vi "Get WiFi Info.vi"(8 "Error In":errorcluster, 11 "LINX Resource":T2={"IO"=enum."Remote", "Interface"=enum."Serial", "LINX Device Config"={"Interface"=enum."Serial", "COM Port"="COM13", "TCP Configuration"={"IP Address"="", "Port"=0}, "Device Family"=1, "Device ID"=1, "Device Name"="myRIO-1900", "TCP Ref"=refnum, "Channels"={"DI"=[0, 1, 2, 3, 4, 5, 6, 7, 8, 9, 10, 11, 12, 13, 14, 15, 16, 17, 18, 19, 20, 21, 22, 23, 24, 25, 26, 27, 28, 29, 30, 31, 32, 33, 34, 35, 36, 37, 38, 39, 40, 41, 42, 43, 44, 45, 46], "DO"=[0, 1, 2, 3, 4, 5, 6, 7, 8, 9, 10, 11, 12, 13, 14, 15, 16, 17, 18, 19, 20, 21, 22, 23, 24, 25, 26, 27, 28, 29, 30, 31, 32, 33, 34, 35, 36, 37, 38, 39, 40, 41, 42, 43, 44, 45, 46], "AI"=[0, 1, 2, 3, 4, 5, 6, 7, 8, 9, 10, 11], "AO"=[], "PWM"=[3, 5, 6, 9, 10], "QE"=[], "UART"=[0, 1], "I2C 2"=[0], "SPI"=[0], "CAN"=[], "Servo"=[], "AI Ref (V)"=0.0, "AI Resolution (Bits)"=0, "AO Ref (V)"=0.0, "AO Resolution (Bits)"=0}}}) -> (0 "Error Out":errorcluster, 1 "TCP Config":T1, 2 "WiFi Info":T7={"SSID"="", "IP Address"="", "Port"=0, "WIFI Security Type"=enum."WPA2 Password", "Password"=""}, 3 "LINX Resource Out":T2={"IO"=enum."Remote", "Interface"=enum."Serial", "LINX Device Config"={"Interface"=enum."Serial", "COM Port"="COM13", "TCP Configuration"={"IP Address"="", "Port"=0}, "Device Family"=1, "Device ID"=1, "Device Name"="myRIO-1900", "TCP Ref"=refnum, "Channels"={"DI"=[0, 1, 2, 3, 4, 5, 6, 7, 8, 9, 10, 11, 12, 13, 14, 15, 16, 17, 18, 19, 20, 21, 22, 23, 24, 25, 26, 27, 28, 29, 30, 31, 32, 33, 34, 35, 36, 37, 38, 39, 40, 41, 42, 43, 44, 45, 46], "DO"=[0, 1, 2, 3, 4, 5, 6, 7, 8, 9, 10, 11, 12, 13, 14, 15, 16, 17, 18, 19, 20, 21, 22, 23, 24, 25, 26, 27, 28, 29, 30, 31, 32, 33, 34, 35, 36, 37, 38, 39, 40, 41, 42, 43, 44, 45, 46], "AI"=[0, 1, 2, 3, 4, 5, 6, 7, 8, 9, 10, 11], "AO"=[], "PWM"=[3, 5, 6, 9, 10], "QE"=[], "UART"=[0, 1], "I2C 2"=[0], "SPI"=[0], "CAN"=[], "Servo"=[], "AI Ref (V)"=0.0, "AI Resolution (Bits)"=0, "AO Ref (V)"=0.0, "AO Resolution (Bits)"=0}}})   [LabVIEW 2019, in "LINXx.lvlib"]
doc: "Lists the WiFi settings currently saved on the device."
uses:
  LINXx.lvlib
  <vilib>/MakerHub/LINX/Private/Device/Type Defs/Wifi Config.ctl
  <vilib>/MakerHub/LINX/Private/Type Defs/WIFI Security Type.ctl
  <vilib>/MakerHub/LINX/Private/Type Defs/LINX Ref.ctl
  <vilib>/MakerHub/LINX/Private/Type Defs/Platform.ctl
  <vilib>/MakerHub/LINX/Private/Type Defs/Interface.ctl
  <vilib>/MakerHub/LINX/Private/Device/Type Defs/LINX Device Config.ctl
  <vilib>/MakerHub/LINX/Private/Device/Type Defs/TCP Config.ctl
  <vilib>/MakerHub/LINX/Private/Device/Type Defs/Channels.ctl
  <vilib>/MakerHub/LINX/Private/Device/Device.lvlib
  <vilib>/MakerHub/LINX/LMH-LINX.lvlib
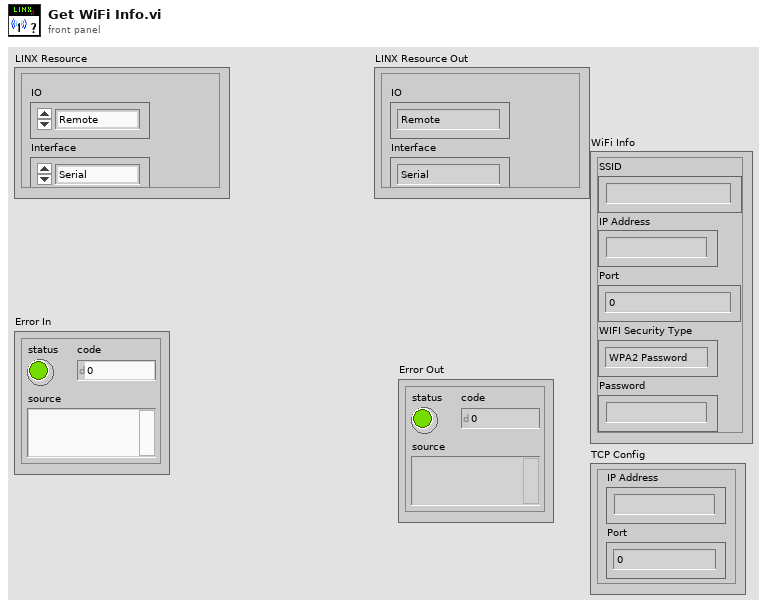
[diagram p1: front panel]
types:
  T1 = typedef "LMH-LINX.lvlib/Device.lvlib/TCP Config.ctl" = cluster{"IP Address":string, "Port":u16}
  T2 = typedef "LMH-LINX.lvlib/LINX Ref.ctl" = cluster{"IO":T3, "Interface":T4, "LINX Device Config":T5}
  T3 = typedef "LMH-LINX.lvlib/Platform.ctl" = enum16{"Remote", "Local"}
  T4 = typedef "LMH-LINX.lvlib/Interface.ctl" = enum16{"Serial", "TCP"}
  T5 = typedef "LMH-LINX.lvlib/Device.lvlib/LINX Device Config.ctl" = cluster{"Interface":T4, "COM Port":refnum<visa-resource-name>, "TCP Configuration":T1, "Device Family":u8, "Device ID":u8, "Device Name":string, "TCP Ref":refnum<k5>, "Channels":T6}
  T6 = typedef "LMH-LINX.lvlib/Channels.ctl" = cluster{"DI":u8[], "DO":u8[], "AI":u8[], "AO":u8[], "PWM":u8[], "QE":u8[], "UART":u8[], "I2C 2":u8[], "SPI":u8[], "CAN":u8[], "Servo":u8[], "AI Ref (V)":dbl, "AI Resolution (Bits)":u8, "AO Ref (V)":dbl, "AO Resolution (Bits)":u8}
  T7 = typedef "LMH-LINX.lvlib/Device.lvlib/Wifi Config.ctl" = cluster{"SSID":string, "IP Address":string, "Port":u16, "WIFI Security Type":T8, "Password":string}
  T8 = typedef "LMH-LINX.lvlib/WIFI Security Type.ctl" = enum8{"None", "WPA2 Password", "WPA2 Key", "WEP40", "WEP104"}
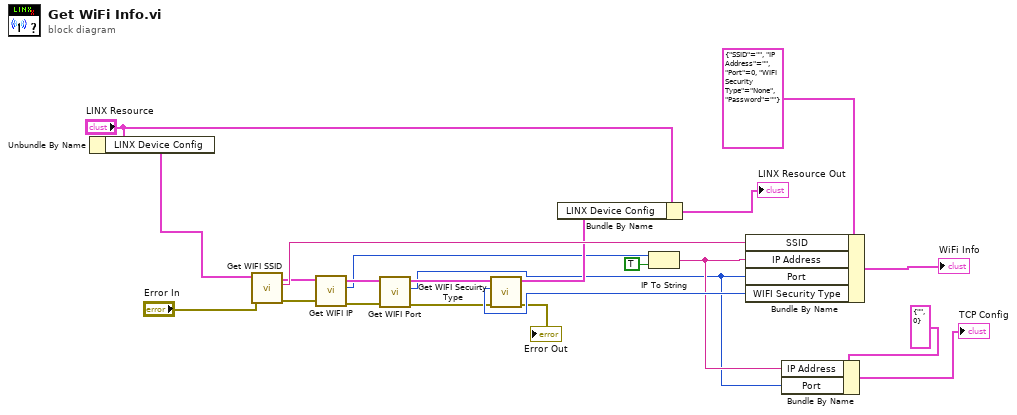
[diagram p0: block diagram]
diagram:
  n1 = Unbundle By Name("LINX Resource") -> ("LINX Device Config"=w10:T5)
  n2 = call <vilib>:"Get WIFI SSID.vi"("Error In"="Error In", "LINX Device Config"=w10) -> ("Error Out"=w15:errorcluster, "SSID"=w21:string, "LINX Device Config"=w17:T5)  [unwired: 7 in]
  n3 = call <vilib>:"Get WIFI IP.vi"("Error In"=w15, "LINX Device Config"=w17) -> ("Error Out"=w14:errorcluster, "Ethernet IP Address"=w1:u32, "LINX Device Config"=w18:T5)  [unwired: 7 in]
  n4 = call <vilib>:"Get WIFI Port.vi"("Error In"=w14, "LINX Device Config"=w18) -> ("Error Out"=w13:errorcluster, "Ethernet Port"=w2:u16, "LINX Device Config"=w19:T5)  [unwired: 7 in]
  n5 = call <vilib>:"Get WIFI Secuirty Type.vi"("Error In"=w13, "LINX Device Config"=w19) -> ("Error Out"=→"Error Out":errorcluster, "LINX Device Config"=w8:T5, "WIFI Security Type"=w20:T8)  [unwired: 7 in]
  n6 = Bundle By Name(cluster="LINX Resource", "LINX Device Config"=w8) -> (→"LINX Resource Out":T2)
  n7 = IP To String(1:TRUE ("dot notation? (F)"), 2:w1) -> (0:w3:string)
  n8 = Bundle By Name(cluster=T7 {"SSID"="", "IP Address"="", "Port"=0, "WIFI Security Type"=enum."None", "Password"=""} ("Wifi Configuration"), "SSID"=w21, "IP Address"=w3, "Port"=w2, "WIFI Security Type"=w20) -> (→"WiFi Info":T7)
  n9 = Bundle By Name(cluster=T1 {"IP Address"="", "Port"=0} ("TCP Config"), "IP Address"=w3, "Port"=w2) -> (→"TCP Config":T1)
